vi "Fluence in Area.vi"(0 "Masked Image":T2, 1 "Origin Image":i64[][](array[numeric]), 5 "Energie":dbl, 7 "calibration mm/px":dbl, 9 "Size of region":i32, 11 "error in (no error)":errorcluster) -> (6 "Fluence J/cm^2":dbl, 8 "Energy in Area":dbl, 10 "Max fluence area":T1, 14 "max value":i64, 15 "error out":errorcluster)   [LabVIEW 2020, in "Analyze.lvlib" / "Analyze Fluence.lvclass"]
uses:
  Analyze Fluence.lvclass
  <vilib>/vision/Image Controls.llb/IMAQ Image.ctl
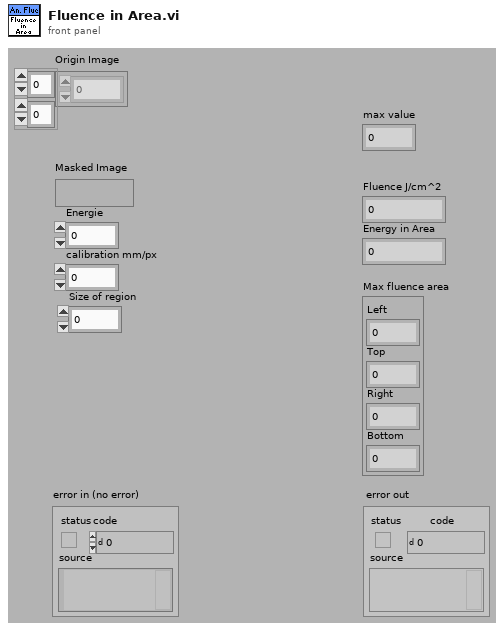
[diagram p1: front panel]
types:
  T1 = cluster{"Left":i32, "Top":i32, "Right":i32, "Bottom":i32}
  T2 = typedef "IMAQ Image.ctl" = refnum<image>
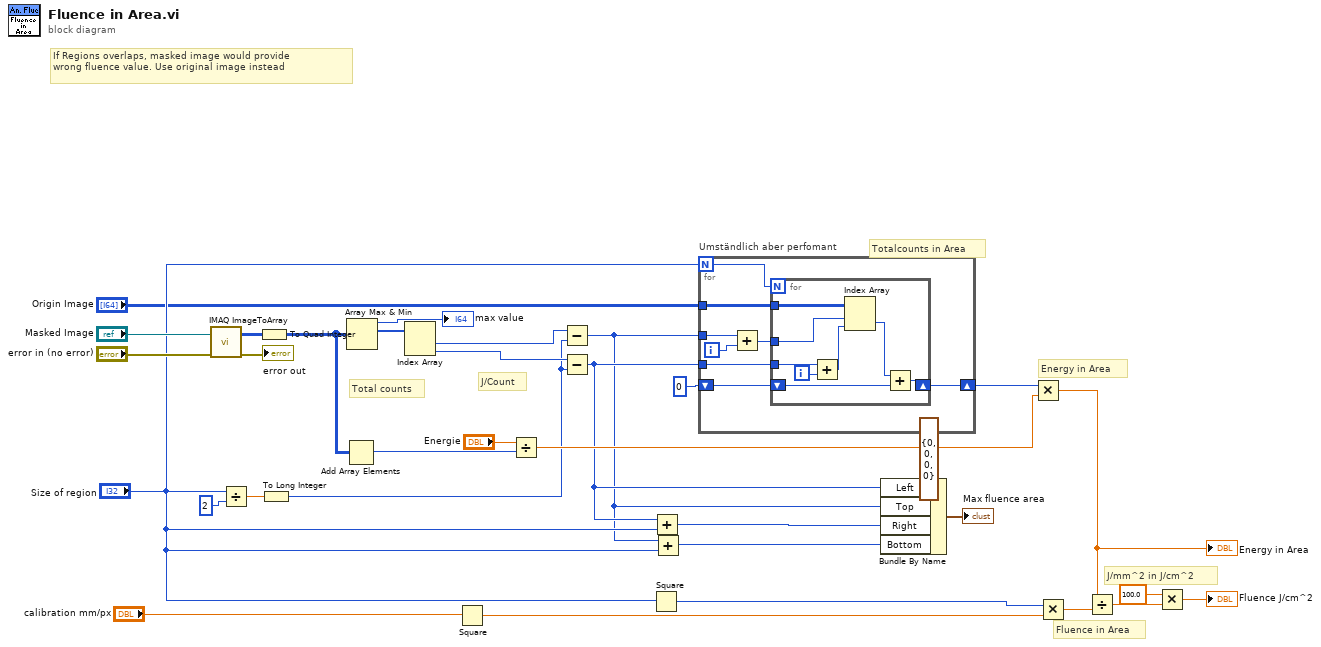
[diagram p0: block diagram]
diagram:
  # "If Regions overlaps, masked image would provide \nwrong fluence value. Use original image instead"
  # "J/mm^2 in J/cm^2"
  # "Fluence in Area"
  # "Totalcounts in Area"
  # "Energy in Area"
  # "J/Count"
  # "Total counts"
  n1 = call "IMAQ ImageToArray"("error in (no error)"="error in (no error)", "Image"="Masked Image") -> ("error out"=→"error out":errorcluster, "Image Pixels (I16)"=w9:i16[][])  [unwired: 2 in, 3 out]
  n2 = Divide(x="Size of region", y=u16 2) -> (x/y=w29:dbl)
  n3 = To Quad Integer(1:w9) -> (0:w8:i64[][])
  n4 = To Long Integer(number=w29) -> (32bit integer=w20:i32)
  n5 = Add Array Elements(numeric array=w8) -> (sum=w18:i64)
  n6 = Array Max & Min(array=w8) -> (max value=→"max value":i64, max index (indices)=w33:i32[])  [unwired: 2 out]
  n7 = Index Array(array=w33) -> (element #1=w30:i32, element #2=w28:i32)  [unwired: 2 in]
  n8 = Square(x="calibration mm/px") -> (x^2=w25:dbl)
  n9 = Divide(x="Energie", y=w18) -> (x/y=w27:dbl)
  n10 = Subtract(x=w30, y=w20) -> (x-y=w1:i32)
  n11 = Subtract(x=w28, y=w20) -> (x-y=w6:i32)
  n12 = Square(x="Size of region") -> (x^2=w24:i32)
  n13 = Add(x=w6, y="Size of region") -> (x+y=w16:i32)
  n14 = Add(x=w1, y="Size of region") -> (x+y=w17:i32)
  n15 = for "Umständlich aber perfomant" {
    N: "Size of region" -> [w34]
    tunnel: w1 -> [w40]
    tunnel: w6 -> [w41]
    shift-right: [w38] -> w3
    shift-left: i64 0 -> [w39]
    tunnel: "Origin Image" -> [w37]
    i -> [w35]
    n16 = Add(x=w40, y=w35) -> (x+y=w36:i32)
    n17 = for {
      N: w34 -> [_]
      tunnel: w41 -> [w45]
      tunnel: w36 -> [w49]
      shift-right: [w43] -> w38
      shift-left: w39 -> [w48]
      tunnel: w37 -> [w47]
      i -> [w46]
      n18 = Add(x=w45, y=w46) -> (x+y=w44:i32)
      n19 = Index Array(array=w47, index (row)=w49, index (col)=w44) -> (element=w42:i64)
      n20 = Add(x=w42, y=w48) -> (x+y=w43:i64)
    }
  }
  n21 = Bundle By Name(cluster=T1 {"Left"=0, "Top"=0, "Right"=0, "Bottom"=0} ("Rectangle"), "Left"=w6, "Top"=w1, "Right"=w16, "Bottom"=w17) -> (→"Max fluence area":T1)
  n22 = Multiply(x=w3, y=w27) -> (x*y=w19:dbl)
  "Energy in Area" <- w19
  n23 = Multiply(x=w24, y=w25) -> (x*y=w23:dbl)
  n24 = Divide(x=w19, y=w23) -> (x/y=w15:dbl)
  n25 = Multiply(x=100.0, y=w15) -> (x*y=→"Fluence J/cm^2":dbl)
